vi "Valves To Num.vi"(8 "valve 14":bool=TRUE, 9 "valve 13":bool=TRUE, 10 "valve 12":bool=TRUE, 11 "valves 1-11":T1(radio)=enum."Vlv_1") -> (3 "Numeric":u32)   [LabVIEW 2020]
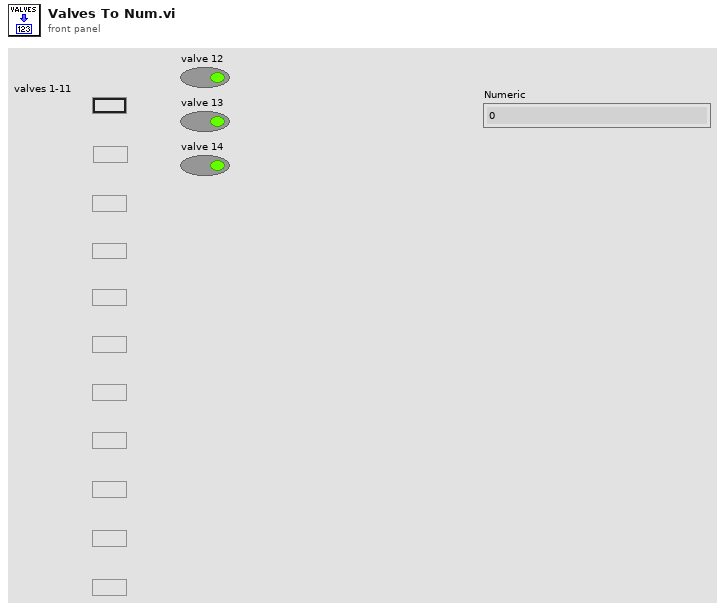
[diagram p1: front panel]
types:
  T1 = enum32{"No Selection", "Vlv_1", "Vlv_1 2", "Vlv_1 3", "Vlv_1 4", "Vlv_1 5", "Vlv_1 6", "Vlv_1 7", "Vlv_1 8", "Vlv_1 9", "Vlv_1 12", "Vlv_1 13"}
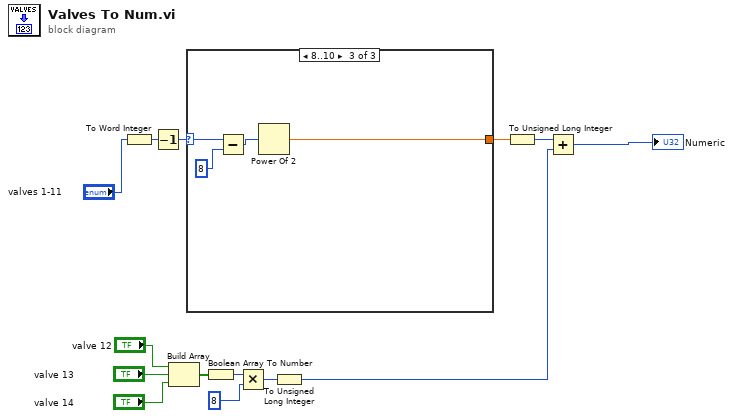
[diagram p0: block diagram]
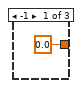
[diagram p2: hidden frame]
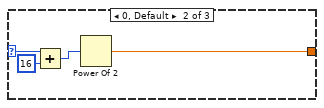
[diagram p3: hidden frame]
diagram:
  n1 = To Word Integer(number="valves 1-11") -> (16bit integer=w12:i16)
  n2 = Decrement(x=w12) -> (x-1=w14:i16)
  n3 = Build Array("valve 12", "valve 13", "valve 14") -> (w8:bool[])
  n4 = case shown="8..10" w14 {
    selector: w14 -> [_ w19 w22]
    tunnel: [0.0 w16 w23] -> w4
    frame -1 {
    }
    frame 0, Default {
      n5 = Add(x=w19, y=i16 16) -> (x+y=w18:i16)
      n6 = Power Of 2(x=w18) -> (2^x=w16:dbl)
    }
    frame 8..10 {
      n7 = Subtract(x=w22, y=i16 8) -> (x-y=w20:i16)
      n8 = Power Of 2(x=w20) -> (2^x=w23:dbl)
    }
  }
  n9 = Boolean Array To Number(Boolean array=w8) -> (number=w7:u32)
  n10 = Multiply(x=w7, y=u32 8) -> (x*y=w5:u32)
  n11 = To Unsigned Long Integer(number=w5) -> (unsigned 32bit integer=w2:u32)
  n12 = To Unsigned Long Integer(number=w4) -> (unsigned 32bit integer=w3:u32)
  n13 = Add(x=w3, y=w2) -> (x+y=→"Numeric":u32)
